vi "PH_DataViewer.get data to modify.vi"(0 "i ref in":refnum<vi>, 3 "ms timeout (10000)":i32=10000, 5 "error in (no error)":errorcluster) -> (14 "i ref out":refnum<vi>, 16 "i attribute":T1, 17 "timed out":bool, 19 "error out":errorcluster)   [LabVIEW 2014, in "PH_DataViewer.lvlib"]
doc: "Reads the attribute data of the object after the access to the data has been locked by the \"acquire\" method. If the attribute data has been locked already, this methods waits until the attribute data is unlocked or there is a timeout.\n\nThe attribute data must be unlocked using the methods \"release\" or \"set modified data\".\n\nLicense Agreement for this software:\n\nCopyright (C)\nGesellschaft für Schwerionenforschung, GSI\nPlanckstr. 1\n64291 Darmstadt\nGermany\n\nContact: D.Beck@gsi.de \n\nThis program is free software; you can redistribute it and/or modify it under the terms of the GNU General Public License as published by the Free Software Foundation; either version 2 of the license, or (at your option) any later version.\n\nThis program is distributed in the hope that it will be useful, but WITHOUT ANY WARRANTY; without even the implied warranty of MERCHANTABILITY or FITNESS FOR A PARTICULAR PURPOSE. See the GNU General License for more details (http://www.gnu.org).\n\nGesellschaft für Schwerionenforschung, GSI\nPlanckstr. 1, 64291 Darmstadt, Germany\nFor all questions and ideas contact: M.Richter@gsi.de, H.Brand@gsi.de or D.Beck@gsi.de.\nLast update: 17-JUN-2004"
uses:
  PH_DataViewer.lvlib
  PH_DataViewer.i attribute.ctl
  CSCore/CSObj/CSObj.lvlib
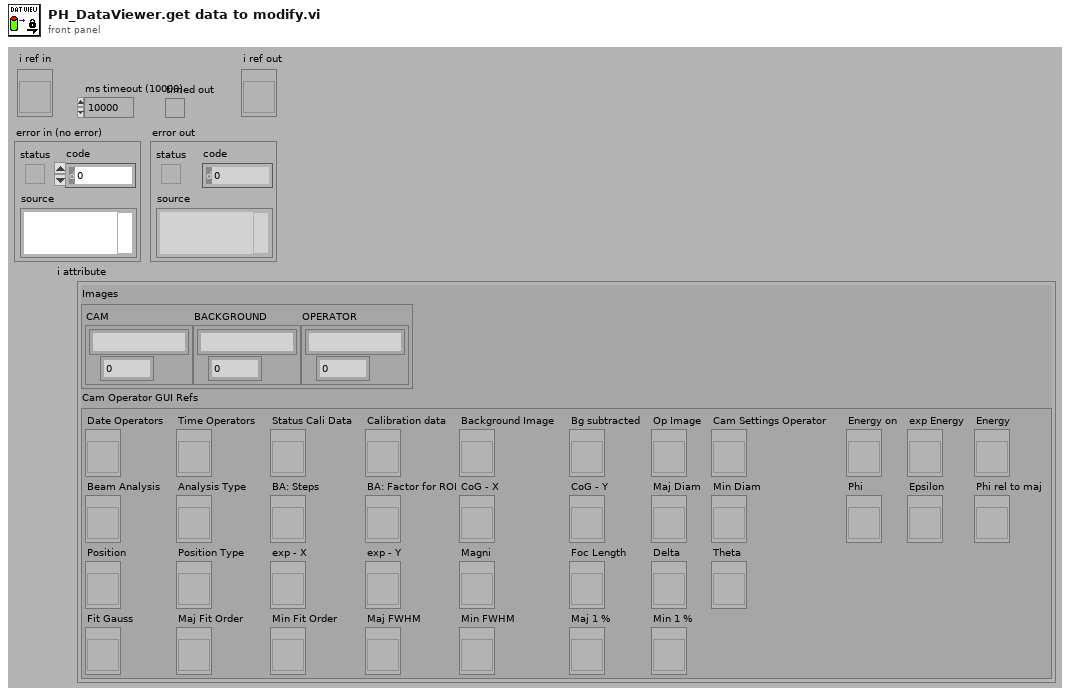
[diagram p1: front panel]
types:
  T1 = typedef "PH_DataViewer.lvlib/PH_DataViewer.i attribute.ctl" = cluster{"Images":cluster{"CAM":cluster{string, u32}, "BACKGROUND":cluster{string, u32}, "OPERATOR":cluster{string, u32}}, "Cam Operator GUI Refs":cluster{"Date Operators":refnum<vi>, "Time Operators":refnum<vi>, "Status Cali Data":refnum<vi>, "Calibration data":refnum<vi>, "Background Image":refnum<vi>, "Bg subtracted":refnum<vi>, "Op Image":refnum<vi>, "Cam Settings Operator":refnum<vi>, "Energy on":refnum<vi>, "exp Energy":refnum<vi>, "Energy":refnum<vi>, "Beam Analysis":refnum<vi>, "Analysis Type":refnum<vi>, "BA: Steps":refnum<vi>, "BA: Factor for ROI":refnum<vi>, "CoG - X":refnum<vi>, "CoG - Y":refnum<vi>, "Maj Diam":refnum<vi>, "Min Diam":refnum<vi>, "Phi":refnum<vi>, "Epsilon":refnum<vi>, "Phi rel to maj":refnum<vi>, "Position":refnum<vi>, "Position Type":refnum<vi>, "exp - X":refnum<vi>, "exp - Y":refnum<vi>, "Magni":refnum<vi>, "Foc Length":refnum<vi>, "Delta":refnum<vi>, "Theta":refnum<vi>, "Fit Gauss":refnum<vi>, "Maj Fit Order":refnum<vi>, "Min Fit Order":refnum<vi>, "Maj FWHM":refnum<vi>, "Min FWHM":refnum<vi>, "Maj 1 %":refnum<vi>, "Min 1 %":refnum<vi>}}
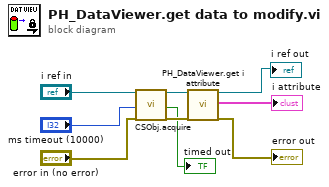
[diagram p0: block diagram]
diagram:
  n1 = call "CSObj.acquire.vi"("i ref in"="i ref in", "ms timeout (10000)"="ms timeout (10000)", "error in (no error)"="error in (no error)") -> ("i ref out"=w8:refnum<vi>, "timed out"=→"timed out":bool, "error out"=w5:errorcluster)  [unwired: 14 in]
  n2 = call "PH_DataViewer.get i attribute.vi"("i ref in"=w8, "error in (no error)"=w5) -> ("i ref out"=→"i ref out":refnum<vi>, "i attribute"=→"i attribute":T1, "error out"=→"error out":errorcluster)  [unwired: 15 in]
